vi "Configure Trigger (I2C).vi"(0 "VISA resource name":refnum<visa-resource-name>, 1 "Address":T2={"Address Mode (0: 7 Bit)"=0, "Address Value (XXXXXXX)"="XXXXXXX"} {"Address Mode (0: 7 Bit)" items=["7 Bit", "10 Bit"]}, 2 "Data":T1={"Data Size (1)"=1, "Data Value (XXXXXXXX)"="XXXXXXXX"}, 5 "Trigger Source (9: Bus 1)":u16(ring)=9 items=["Bus 1"=9, "Bus 2"=10, "Bus 3"=11, "Bus 4"=12], 7 "Trigger Condition (0: Start)":u16(ring) items=["Start", "Stop", "Repeat Start", "Ack Miss", "Address", "Data", "Address & Data"], 9 "Direction (0: Read)":u16(ring) items=["Read", "Write", "Read or Write"], 11 "error in (no error)":errorcluster) -> (4 "VISA resource name out":refnum<visa-resource-name>, 15 "error out":errorcluster)   [LabVIEW 2009, in "Tektronix DPO MSO 2000 4000 Series.lvlib"]
doc: "Configures I2C trigger settings for an oscilloscope."
uses:
  <instrlib>/Tektronix DPO MSO 2000 4000 Series/Tektronix DPO MSO 2000 4000 Series.lvlib
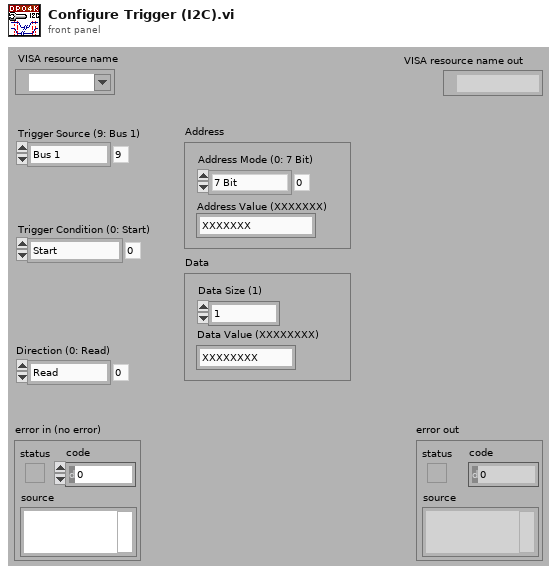
[diagram p1: front panel]
types:
  T1 = cluster{"Data Size (1)":i32, "Data Value (XXXXXXXX)":string}
  T2 = cluster{"Address Mode (0: 7 Bit)":u16, "Address Value (XXXXXXX)":string}
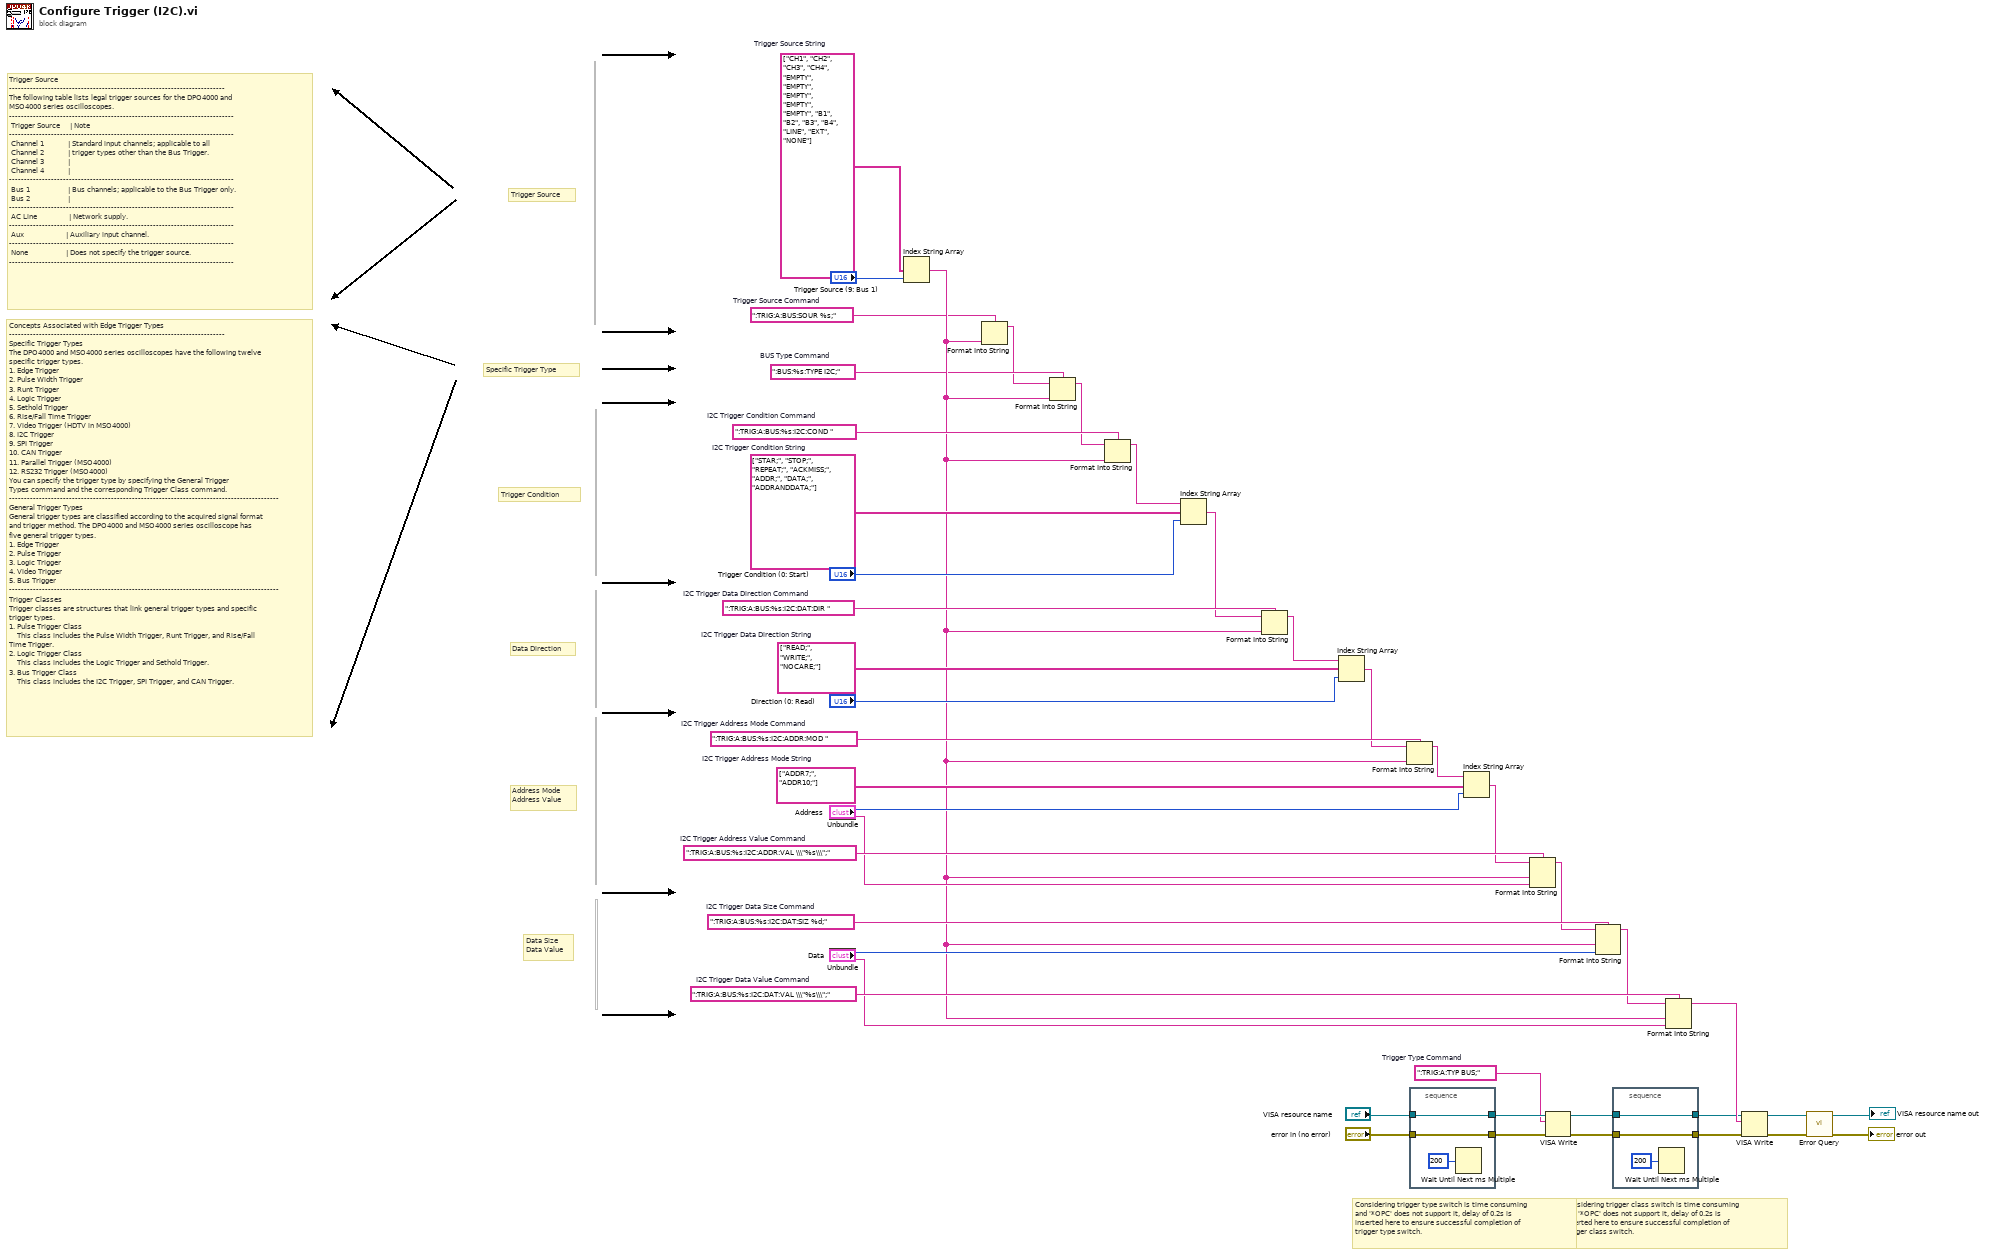
[diagram p0: block diagram]
diagram:
  w21 = string[] ["CH1", "CH2", "CH3", "CH4", "EMPTY", "EMPTY", "EMPTY", "EMPTY", "EMPTY", "B1", "B2", "B3", "B4", "LINE", "EXT", "NONE"]  # Trigger Source String
  w18 = ":TRIG:A:BUS:SOUR %s;"  # Trigger Source Command
  w23 = ":TRIG:A:BUS:%s:I2C:DAT:VAL \\\"%s\\\";"  # I2C Trigger Data Value Command
  w25 = ":TRIG:A:BUS:%s:I2C:DAT:SIZ %d;"  # I2C Trigger Data Size Command
  w28 = ":TRIG:A:BUS:%s:I2C:ADDR:VAL \\\"%s\\\";"  # I2C Trigger Address Value Command
  w30 = string[] ["ADDR7;", "ADDR10;"]  # I2C Trigger Address Mode String
  w32 = ":TRIG:A:BUS:%s:I2C:ADDR:MOD "  # I2C Trigger Address Mode Command
  w35 = string[] ["READ;", "WRITE;", "NOCARE;"]  # I2C Trigger Data Direction String
  w37 = ":TRIG:A:BUS:%s:I2C:DAT:DIR "  # I2C Trigger Data Direction Command
  w39 = string[] ["STAR;", "STOP;", "REPEAT;", "ACKMISS;", "ADDR;", "DATA;", "ADDRANDDATA;"]  # I2C Trigger Condition String
  w40 = ":TRIG:A:BUS:%s:I2C:COND "  # I2C Trigger Condition Command
  w19 = ":BUS:%s:TYPE I2C;"  # BUS Type Command
  w44 = ":TRIG:A:TYP BUS;"  # Trigger Type Command
  # "Concepts Associated with Edge Trigger Types\n------------------------------------------------------------------------\nSpecific Trigger Types\nThe DPO4000 and MSO4000 series oscilloscopes have the following twelve specific trigger types.\n1. Edge Trigger\n2. Pulse Width Trigger\n3. Runt Trigger\n4. Logic Trigger\n5. Sethold Trigger\n6. Rise/Fall Time Trigger\n7. Video Trigger (HDTV in MSO4000)\n8. I2C Trigger\n9. SPI Trigger\n10. CAN Trigger\n11. Parallel Trigger (MSO4000)\n12. RS232 Trigger (MSO4000)\nYou can specify the trigger type by specifying the General Trigger \nTypes command and the corresponding Trigger Class command.\n------------------------------------------------------------------------------------------\nGeneral Trigger Types \nGeneral trigger types are classified according to the acquired signal format and trigger method. The DPO4000 and MSO4000 series oscilloscope has five general trigger types.\n1. Edge Trigger\n2. Pulse Trigger\n3. Logic Trigger\n4. Video Trigger\n5. Bus Trigger\n------------------------------------------------------------------------------------------\nTrigger Classes\nTrigger classes are structures that link general trigger types and specific trigger types.\n1. Pulse Trigger Class\n    This class includes the Pulse Width Trigger, Runt Trigger, and Rise/Fall Time Trigger.\n2. Logic Trigger Class\n    This class includes the Logic Trigger and Sethold Trigger.\n3. Bus Trigger Class\n    This class includes the I2C Trigger, SPI Trigger, and CAN Trigger."
  # "Trigger Source\n------------------------------------------------------------------------\nThe following table lists legal trigger sources for the DPO4000 and MSO4000 series oscilloscopes.\n---------------------------------------------------------------------------\n Trigger Source     | Note                                                           \n---------------------------------------------------------------------------\n Channel 1            | Standard input channels; applicable to all      \n Channel 2            | trigger types other than the Bus Trigger.         \n Channel 3            |     \n Channel 4            |\n---------------------------------------------------------------------------\n Bus 1                   | Bus channels; applicable to the Bus Trigger only.\n Bus 2                   | \n---------------------------------------------------------------------------\n AC Line                | Network supply.\n---------------------------------------------------------------------------\n Aux                     | Auxiliary input channel.\n---------------------------------------------------------------------------\n None                   | Does not specify the trigger source.\n---------------------------------------------------------------------------"
  # "Considering trigger class switch is time consuming\nand '*OPC' does not support it, delay of 0.2s is \ninserted here to ensure successful completion of\ntrigger class switch."
  # "Data Size\nData Value"
  # "Address Mode\nAddress Value"
  # "Data Direction"
  # "Trigger Condition"
  # "Specific Trigger Type"
  # "Trigger Source"
  # "Considering trigger type switch is time consuming\nand '*OPC' does not support it, delay of 0.2s is \ninserted here to ensure successful completion of\ntrigger type switch."
  n1 = Unbundle("Address") -> ("Address Mode (0: 7 Bit)"=w29:u16, "Address Value (XXXXXXX)"=w27:string)
  n2 = Unbundle("Data") -> ("Data Size (1)"=w24:i32, "Data Value (XXXXXXXX)"=w22:string)
  n3 = Index String Array(1:"Trigger Source (9: Bus 1)", 2:w21) -> (0:w20:string)  [unwired: 1 in]
  n4 = Format Into String(format string=w18, w20) -> (resulting string=w17:string)  [unwired: 2 in, 1 out]
  n5 = Format Into String(format string=w19, initial string=w17, w20) -> (resulting string=w16:string)  [unwired: 1 in, 1 out]
  n6 = Format Into String(format string=w40, initial string=w16, w20) -> (resulting string=w15:string)  [unwired: 1 in, 1 out]
  n7 = Index String Array(1:"Trigger Condition (0: Start)", 2:w39, 3:w15) -> (0:w14:string)
  n8 = Format Into String(format string=w37, initial string=w14, w20) -> (resulting string=w36:string)  [unwired: 1 in, 1 out]
  n9 = Index String Array(1:"Direction (0: Read)", 2:w35, 3:w36) -> (0:w13:string)
  n10 = Format Into String(format string=w32, initial string=w13, w20) -> (resulting string=w31:string)  [unwired: 1 in, 1 out]
  n11 = stacked-sequence {
    tunnel: "VISA resource name" -> [w48]
    tunnel: [w48] -> w46
    tunnel: "error in (no error)" -> [w47]
    tunnel: [w47] -> w45
    frame #0 {
      n12 = Wait Until Next ms Multiple(millisecond multiple=u32 200) -> ()  [unwired: 1 out]
    }
  }
  n13 = Index String Array(1:w29, 2:w30, 3:w31) -> (0:w9:string)
  n14 = Format Into String(format string=w28, initial string=w9, w20, w27) -> (resulting string=w12:string)  [unwired: 1 in, 1 out]
  n15 = VISA Write(VISA resource name=w46, write buffer=w44, error in (no error)=w45) -> (VISA resource name out=w43:refnum<visa-resource-name>, error out=w42:errorcluster)  [unwired: 1 out]
  n16 = Format Into String(format string=w25, initial string=w12, w20, w24) -> (resulting string=w11:string)  [unwired: 1 in, 1 out]
  n17 = stacked-sequence {
    tunnel: w43 -> [w51]
    tunnel: [w51] -> w8
    tunnel: w42 -> [w50]
    tunnel: [w50] -> w7
    frame #0 {
      n18 = Wait Until Next ms Multiple(millisecond multiple=u32 200) -> ()  [unwired: 1 out]
    }
  }
  n19 = Format Into String(format string=w23, initial string=w11, w20, w22) -> (resulting string=w10:string)  [unwired: 1 in, 1 out]
  n20 = VISA Write(VISA resource name=w8, write buffer=w10, error in (no error)=w7) -> (VISA resource name out=w6:refnum<visa-resource-name>, error out=w5:errorcluster)  [unwired: 1 out]
  n21 = call <instrlib>:"Error Query.vi"("error in (no error)"=w5, "VISA resource name"=w6) -> ("error out"=→"error out":errorcluster, "VISA resource name out"=→"VISA resource name out":refnum<visa-resource-name>)  [unwired: 6 in, 2 out]
